vi "read inputs from fpga.vi"(7 "data table in in":T7, 8 "error in (no error)":errorcluster, 9 "diagnostics":T5[](array[typedef]), 10 "inputs":T2[](array[typedef]), 11 "Refnum in":T1) -> (0 "error out":errorcluster, 3 "data table out":T7)   [LabVIEW 2013, in "Profibus Module runtime.lvclass"]
uses:
  Profibus Module runtime.lvclass
  <vilib>/NI/Tag Bus/table/data table.ctl
  profibus diagnostics reporting.ctl
  configuration/error throw specification.ctl
  profibus slave configuration.ctl
  profibus mapping configuration.ctl
  <vilib>/NI/Tag Bus/tag/Data Type.ctl
  dynamic profibus/fpga reference.ctl
  dynamic profibus/dynamic profibus.lvlib
  <vilib>/NI/Tag Bus/table/data table.lvlib
  configuration/Profibus Module configuration.lvclass
  <vilib>/NI/Tag Bus/tag/tag descriptor.lvclass
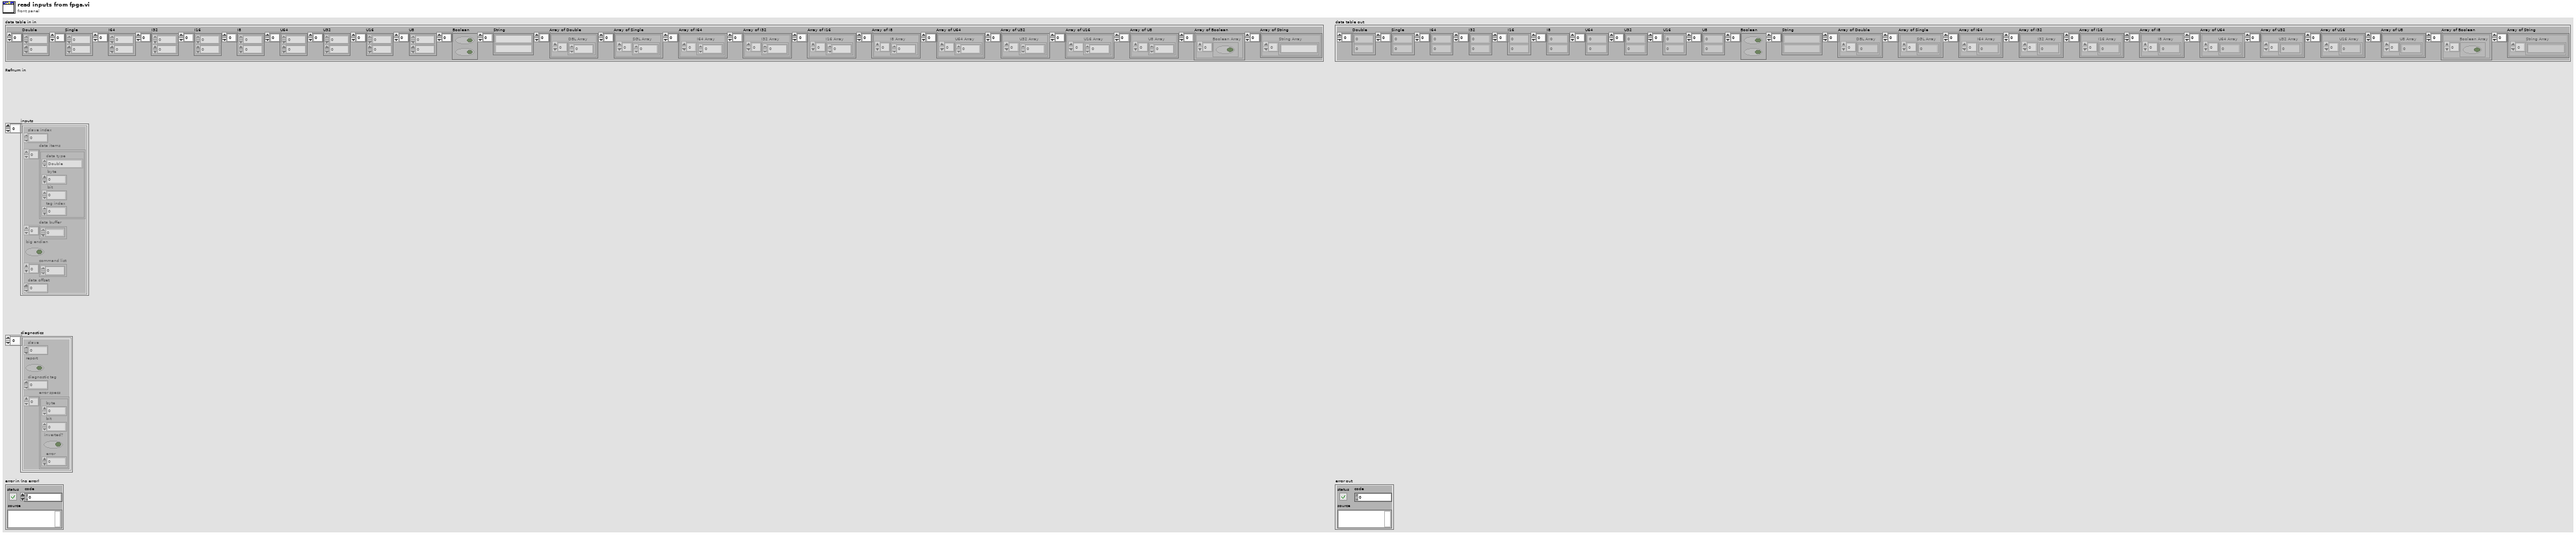
[diagram p1: front panel]
types:
  T1 = typedef "dynamic profibus.lvlib/fpga reference.ctl" = refnum<k20>
  T2 = typedef "Profibus Module runtime.lvclass/profibus slave configuration.ctl" = cluster{"slave index":i8, "data items":T3[], "data buffer":u8[], "big endian":bool, "command list":u32[], "data offset":u8}
  T3 = typedef "Profibus Module runtime.lvclass/profibus mapping configuration.ctl" = cluster{"data type":T4, " byte":i32, " bit":i32, "tag index":i32}
  T4 = typedef "tag bus.lvlib/tag descriptor.lvclass/Data Type.ctl" = enum16{"Double", "Single", "I64", "I32", "I16", "I8", "U64", "U32", "U16", "U8", "Boolean", "String", "Array of Double", "Array of Single", "Array of I64", "Array of I32", "Array of I16", "Array of I8", "Array of U64", "Array of U32", "Array of U16", "Array of U8", "Array of Boolean", "Array of String"}
  T5 = typedef "Profibus Module runtime.lvclass/profibus diagnostics reporting.ctl" = cluster{"slave":i8, "report":bool, "diagnostic tag":i32, "error specs":T6[]}
  T6 = typedef "Profibus Module configuration.lvclass/error throw specification.ctl" = cluster{"byte":i32, "bit":i32, "inverted?":bool, "error":i32}
  T7 = typedef "tag bus.lvlib/data table.lvlib/data table.ctl" = cluster{"Double":dbl[], "Single":sgl[], "I64":i64[], "I32":i32[], "I16":i16[], "I8":i8[], "U64":u64[], "U32":u32[], "U16":u16[], "U8":u8[], "Boolean":bool[], "String":string[], "Array of Double":cluster{"DBL Array":dbl[]}[], "Array of Single":cluster{"SGL Array":sgl[]}[], "Array of I64":cluster{"I64 Array":i64[]}[], "Array of I32":cluster{"I32 Array":i32[]}[], "Array of I16":cluster{"I16 Array":i16[]}[], "Array of I8":cluster{"I8 Array":i8[]}[], "Array of U64":cluster{"U64 Array":u64[]}[], "Array of U32":cluster{"U32 Array":u32[]}[], "Array of U16":cluster{"U16 Array":u16[]}[], "Array of U8":cluster{"U8 Array":u8[]}[], "Array of Boolean":cluster{"Boolean Array":bool[]}[], "Array of String":cluster{"String Array":string[]}[]}
  T8 = typedef "dynamic profibus.lvlib/profibus master transmit header.ctl" = enum8{"Error", "Input", "Diagnostic", "input size", "output size", "many inputs"}
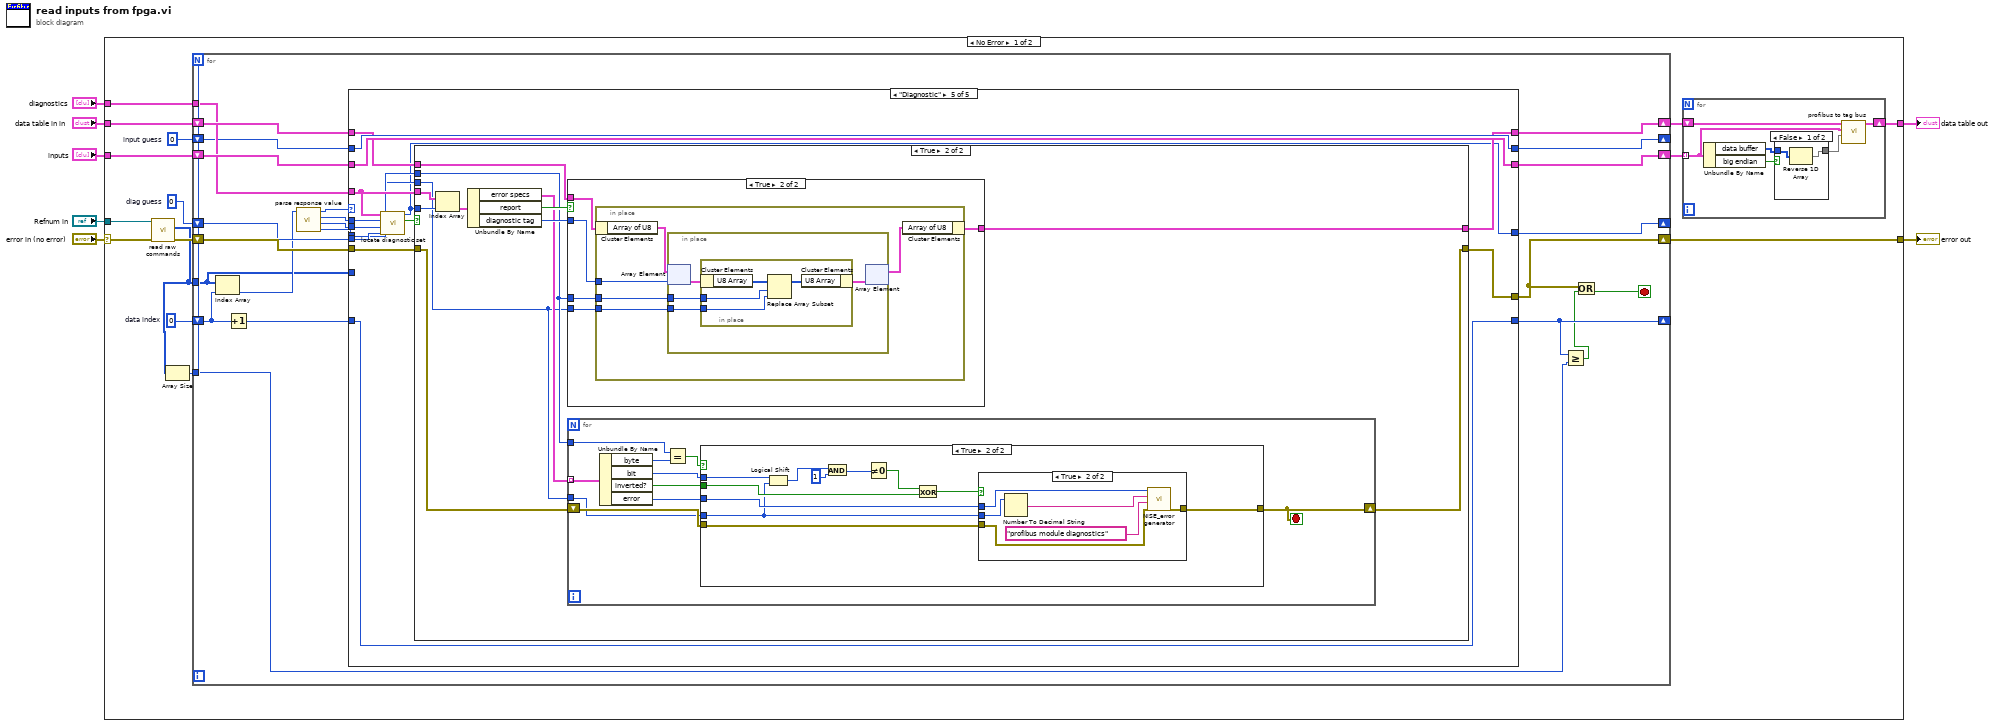
[diagram p0: block diagram]
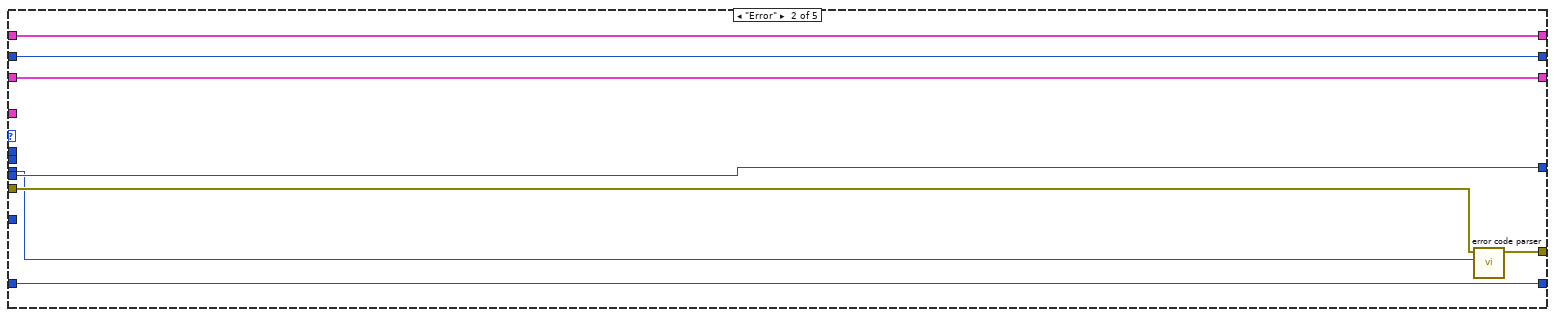
[diagram p3: hidden frame]
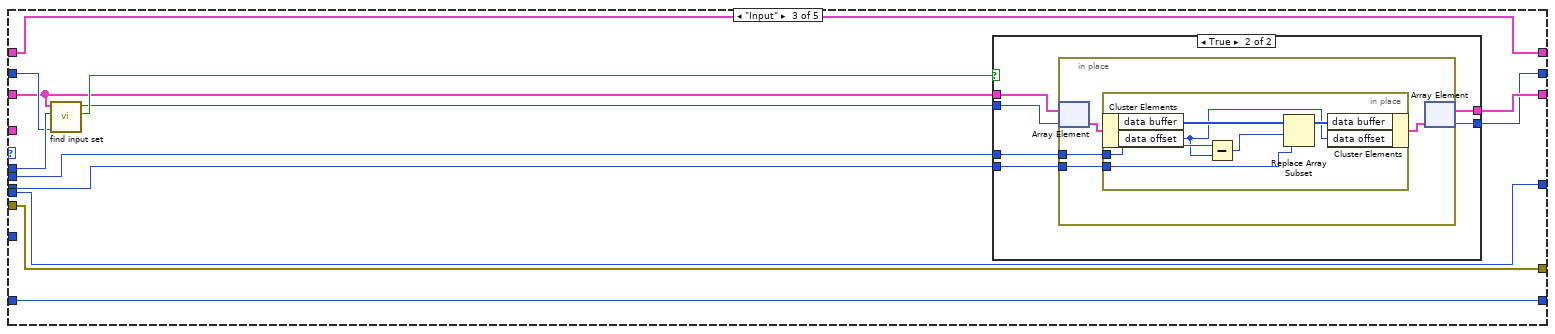
[diagram p4: hidden frame]
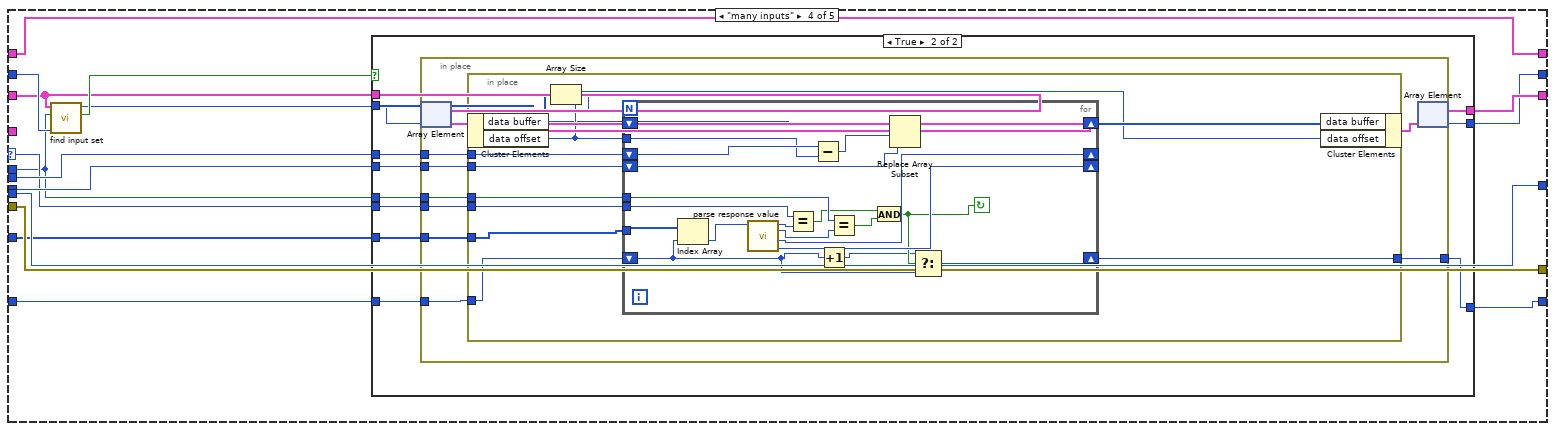
[diagram p6: hidden frame]
diagram:
  n1 = case shown="No Error" "error in (no error)" {
    selector: "error in (no error)" -> [w12 w247]
    tunnel: "inputs" -> [w20 _]
    tunnel: [w22 w246] -> w7
    tunnel: [w16 w247] -> w6
    tunnel: "Refnum in" -> [w13 _]
    tunnel: "diagnostics" -> [w21 _]
    tunnel: "data table in in" -> [w19 w246]
    frame No Error {
      w10 = 0  # data index
      w14 = 0  # diag guess
      w15 = 0  # input guess
      n2 = call "read raw commands.vi"("error in"=w12, "profibus reference"=w13) -> ("error out"=w11:errorcluster, "Data"=w9:u32[])  [unwired: 7 in, 1 out]
      n3 = Array Size(array=w9) -> (size(s)=w8:i32)
      n4 = for {
        N: w8 -> [_]
        tunnel: w21 -> [w40]
        shift-right: [w43] -> w17
        shift-left: w20 -> [w44]
        shift-right: [w42] -> w18
        shift-left: w19 -> [w41]
        shift-right: [w39] -> w16
        shift-left: w11 -> [w45]
        shift-right: [w37] -> _
        shift-left: w15 -> [w38]
        shift-right: [w35] -> _
        shift-left: w14 -> [w36]
        tunnel: w9 -> [w27]
        shift-right: [w25] -> _
        shift-left: w10 -> [w30]
        tunnel: w8 -> [w24]
        stop <- w26 stop-if-true
        n5 = Index Array(array=w27, index=w30) -> (element=w28:u32)
        n6 = Increment(x=w30) -> (x+1=w29:i32)
        n7 = call "parse response value.vi"("Element"=w28) -> ("data"=w31:u8, "index"=w32:u8, "device"=w33:u8, "header"=w34:T8)  [unwired: 7 in]
        n8 = case shown="\"Diagnostic\"" w34 {
          selector: w34 -> [_ _ _ w92 _]
          tunnel: w45 -> [w49 w54 w71 w105 w167]
          tunnel: [w49 w55 w71 w105 w168] -> w39
          tunnel: w33 -> [_ _ w70 w91 w171]
          tunnel: w31 -> [_ w53 w62 w97 w163]
          tunnel: w44 -> [w51 w59 w67 w102 w174]
          tunnel: [w51 w59 w66 w101 w174] -> w43
          tunnel: w32 -> [_ _ w63 w98 w164]
          tunnel: [w50 w58 w72 w106 w169] -> w42
          tunnel: w41 -> [w50 w58 w72 w106 w170]
          tunnel: w40 -> [_ _ _ _ w165]
          tunnel: w38 -> [w48 w57 w69 w104 w173]
          tunnel: [w48 w57 w64 w99 w173] -> w37
          tunnel: w36 -> [w47 w56 w61 w96 w172]
          tunnel: [w47 w56 w61 w96 w162] -> w35
          tunnel: w29 -> [w46 w52 w60 w93 w161]
          tunnel: [w46 w52 w60 w94 w161] -> w25
          tunnel: w27 -> [_ _ _ w95 _]
          frame "input size", "output size" {
          }
          frame "Error" {
            n9 = call "error code parser.vi"("Error"=w54, "Status"=w53) -> ("Error out"=w55:errorcluster)  [unwired: 7 in]
          }
          frame "Input" {
            n10 = call "find input set.vi"("input guess in"=w69, "device"=w70, "inputs"=w67) -> ("found?"=w68:bool, "index out"=w65:i32)  [unwired: 7 in]
            n11 = case shown="True" w68 {
              tunnel: w67 -> [w74 w80]
              tunnel: [w74 w78] -> w66
              tunnel: w65 -> [w73 w79]
              tunnel: [w73 w77] -> w64
              tunnel: w63 -> [_ w76]
              tunnel: w62 -> [_ w75]
              frame False {
              }
              frame True {
                n12 = in-place {
                  in-place-border: w76 -> [w82]
                  in-place-border: w75 -> [w81]
                  n13 = in-place-array #1(w80, w79) -> (w84:T2)
                  n14 = in-place {
                    in-place-border: w82 -> [w87]
                    in-place-border: w81 -> [w88]
                    n15 = in-place-cluster #2(w84) -> ("data buffer"=w90:u8[], "data offset"=w85:u8)
                    n16 = Subtract(x=w87, y=w85) -> (x-y=w86:u8)
                    n17 = Replace Array Subset(array=w90, new element=w88, index=w86) -> (w89:u8[])
                    n18 = in-place-cluster #2("data buffer"=w89, "data offset"=w85) -> (w83:T2)
                  }
                  n19 = in-place-array #1(w83) -> (w78:T2[], w77:i32)
                }
              }
            }
          }
          frame "many inputs" {
            n20 = call "find input set.vi"("input guess in"=w104, "device"=w91, "inputs"=w102) -> ("found?"=w103:bool, "index out"=w100:i32)  [unwired: 7 in]
            n21 = case shown="True" w103 {
              tunnel: w102 -> [w109 w120]
              tunnel: [w109 w118] -> w101
              tunnel: w100 -> [w108 w119]
              tunnel: [w108 w117] -> w99
              tunnel: w98 -> [_ w116]
              tunnel: w97 -> [_ w115]
              tunnel: w95 -> [_ w114]
              tunnel: [w107 w110] -> w94
              tunnel: w93 -> [w107 w113]
              tunnel: w92 -> [_ w112]
              tunnel: w91 -> [_ w111]
              frame False {
              }
              frame True {
                n22 = in-place {
                  in-place-border: w116 -> [w127]
                  in-place-border: w115 -> [w126]
                  in-place-border: w114 -> [w125]
                  in-place-border: w113 -> [w124]
                  in-place-border: w112 -> [w123]
                  in-place-border: w111 -> [w122]
                  in-place-border: [w121] -> w110
                  n23 = in-place-array #3(w120, w119) -> (w129:T2)
                  n24 = in-place {
                    in-place-border: w127 -> [w138]
                    in-place-border: w126 -> [w139]
                    in-place-border: w125 -> [w136]
                    in-place-border: w124 -> [w135]
                    in-place-border: w123 -> [w134]
                    in-place-border: w122 -> [w133]
                    in-place-border: [w132] -> w121
                    n25 = in-place-cluster #4(w129) -> ("data buffer"=w131:u8[], "data offset"=w137:u8)
                    n26 = Array Size(array=w131) -> (size(s)=w130:i32)
                    n27 = for {
                      N: w130 -> [_]
                      tunnel: w137 -> [w155]
                      shift-right: [w159] -> w140
                      shift-left: w131 -> [w160]
                      tunnel: w136 -> [w154]
                      shift-right: [w141] -> w132
                      shift-left: w135 -> [w142]
                      tunnel: w134 -> [w151]
                      tunnel: w133 -> [w149]
                      shift-right: [w148] -> _
                      shift-left: w138 -> [w157]
                      shift-right: [w147] -> _
                      shift-left: w139 -> [w158]
                      stop <- w144 continue-if-true
                      n28 = Index Array(array=w154, index=w142) -> (element=w153:u32)
                      n29 = call "parse response value.vi"("Element"=w153) -> ("data"=w147:u8, "index"=w148:u8, "device"=w150:u8, "header"=w152:T8)  [unwired: 7 in]
                      n30 = Equal?(x=w151, y=w152) -> (x = y?=w145:bool)
                      n31 = Subtract(x=w157, y=w155) -> (x-y=w156:u8)
                      n32 = Increment(x=w142) -> (x+1=w143:i32)
                      n33 = Equal?(x=w149, y=w150) -> (x = y?=w146:bool)
                      n34 = And(x=w145, y=w146) -> (x .and. y?=w144:bool)
                      n35 = Replace Array Subset(array=w160, new element=w158, index=w156) -> (w159:u8[])
                      n36 = Select(t=w143, s=w144, f=w142) -> (s? t:f=w141:i32)
                    }
                    n37 = in-place-cluster #4("data buffer"=w140, "data offset"=w137) -> (w128:T2)
                  }
                  n38 = in-place-array #3(w128) -> (w118:T2[], w117:i32)
                }
              }
            }
          }
          frame "Diagnostic" {
            n39 = call "locate diagnostic set.vi"("guess index"=w172, "device"=w171, "diagnostics"=w165) -> ("found?"=w166:bool, "index"=w162:i32)  [unwired: 7 in]
            n40 = case shown="True" w166 {
              tunnel: [w176 w185] -> w169
              tunnel: w170 -> [w176 w184]
              tunnel: [w175 w179] -> w168
              tunnel: w167 -> [w175 w180]
              tunnel: w165 -> [_ w188]
              tunnel: w162 -> [_ w187]
              tunnel: w164 -> [_ w178]
              tunnel: w163 -> [_ w177]
              frame False {
              }
              frame True {
                n41 = Index Array(array=w188, index=w187) -> (element=w186:T5)
                n42 = Unbundle By Name(w186) -> ("error specs"=w181:T6[], "report"=w183:bool, "diagnostic tag"=w182:i32)
                n43 = case shown="True" w183 {
                  tunnel: w184 -> [w218 w223]
                  tunnel: [w218 w222] -> w185
                  tunnel: w182 -> [_ w221]
                  tunnel: w178 -> [_ w220]
                  tunnel: w177 -> [_ w219]
                  frame False {
                  }
                  frame True {
                    n44 = in-place {
                      in-place-border: w221 -> [w227]
                      in-place-border: w220 -> [w225]
                      in-place-border: w219 -> [w224]
                      n45 = in-place-cluster #5(w223) -> ("Array of U8"=w228:cluster{"U8 Array":u8[]}[])
                      n46 = in-place {
                        in-place-border: w225 -> [w230]
                        in-place-border: w224 -> [w229]
                        n47 = in-place-array #6(w228, w227) -> (w232:cluster{"U8 Array":u8[]})
                        n48 = in-place {
                          in-place-border: w230 -> [w234]
                          in-place-border: w229 -> [w233]
                          n49 = in-place-cluster #7(w232) -> ("U8 Array"=w236:u8[])
                          n50 = Replace Array Subset(array=w236, new element=w233, index=w234) -> (w235:u8[])
                          n51 = in-place-cluster #7("U8 Array"=w235) -> (w231:cluster{"U8 Array":u8[]})
                        }
                        n52 = in-place-array #6(w231) -> (w226:cluster{"U8 Array":u8[]}[])  [unwired: 1 out]
                      }
                      n53 = in-place-cluster #5("Array of U8"=w226) -> (w222:T7)
                    }
                  }
                }
                n54 = for {
                  tunnel: w181 -> [w198] mode=indexing
                  shift-right: [w193] -> w179
                  shift-left: w180 -> [w194]
                  tunnel: w178 -> [w196]
                  tunnel: w177 -> [w190]
                  stop <- w193 stop-if-true
                  n55 = Unbundle By Name(w198) -> ("byte"=w197:i32, "bit"=w192:i32, "inverted?"=w191:bool, "error"=w189:i32)
                  n56 = Equal?(x=w196, y=w197) -> (x = y?=w195:bool)
                  n57 = case shown="True" w195 {
                    tunnel: [w199 w202] -> w193
                    tunnel: w194 -> [w199 w203]
                    tunnel: w192 -> [_ w206]
                    tunnel: w191 -> [_ w205]
                    tunnel: w190 -> [_ w200]
                    tunnel: w189 -> [_ w201]
                    frame False {
                    }
                    frame True {
                      n58 = Logical Shift(y=w206, x=w200) -> (x << y=w210:u8)
                      n59 = And(x=w210, y=u8 1) -> (x .and. y?=w208:u8)
                      n60 = Not Equal To 0?(x=w208) -> (x != 0?=w207:bool)
                      n61 = Exclusive Or(1:w205, 2:w207) -> (0:w204:bool)
                      n62 = case shown="True" w204 {
                        tunnel: w203 -> [w211 w213]
                        tunnel: [w211 w212] -> w202
                        tunnel: w201 -> [_ w215]
                        tunnel: w200 -> [_ w214]
                        frame False {
                        }
                        frame True {
                          n63 = Number To Decimal String(number=w214) -> (decimal integer string=w216:string)  [unwired: 1 in]
                          n64 = call <vilib>:"NISE_error generator.vi"("error in"=w213, "source"="profibus module diagnostics", "append error message"=w216, "error code (0)"=w215) -> ("error out"=w212:errorcluster)  [unwired: 5 in]
                        }
                      }
                    }
                  }
                }
              }
            }
          }
        }
        n65 = Greater Or Equal?(x=w25, y=w24) -> (x >= y?=w23:bool)
        n66 = Or(x=w39, y=w23) -> (x .or. y?=w26:bool)
      }
      n67 = for {
        shift-right: [w242] -> w22
        shift-left: w18 -> [w241]
        tunnel: w17 -> [w237] mode=indexing
        n68 = Unbundle By Name(w237) -> ("data buffer"=w238:u8[], "big endian"=w240:bool)
        n69 = case shown="False" w240 {
          tunnel: [w243 w245] -> w239
          tunnel: w238 -> [w244 w245]
          frame False {
            n70 = Reverse 1D Array(array=w244) -> (reversed array=w243:u8[])
          }
          frame True {
          }
        }
        n71 = call "profibus to tag bus.vi"("Data in"=w239, "slave configuration"=w237, "data table in"=w241) -> ("data table out"=w242:T7)  [unwired: 8 in]
      }
    }
    frame Error {
    }
  }
  "data table out" <- w7
  "error out" <- w6
